vi "Acquire Pulse Result.vi"(8 "error in (no error)":errorcluster, 11 "Pulse Driver in":refnum<class "Pulse Driver.lvclass">) -> (0 "error out":errorcluster, 2 "Pulse acquired":bool, 3 "Pulse Driver out":refnum<class "Pulse Driver.lvclass">)   [LabVIEW 2021, in "Pulse Driver.lvclass"]
uses:
  Pulse Driver.lvclass
  Pulse Driver.lvclass/Pulse Driver.ctl
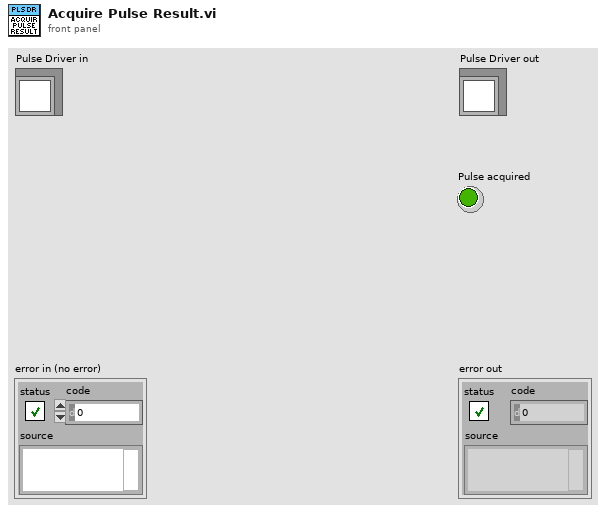
[diagram p1: front panel]
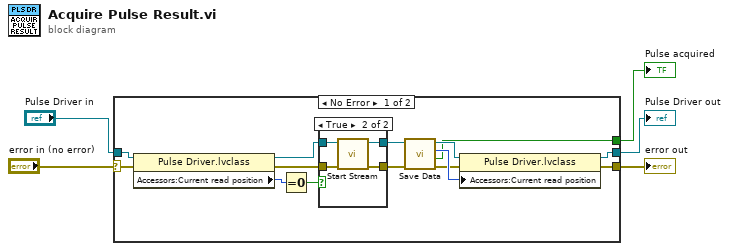
[diagram p0: block diagram]
diagram:
  n1 = case shown="No Error" "error in (no error)" {
    selector: "error in (no error)" -> [w16 w27]
    tunnel: [w8 w27] -> w4
    tunnel: [w12 w26] -> w2
    tunnel: "Pulse Driver in" -> [w15 w26]
    tunnel: [w6 _] -> w1
    frame No Error {
      n2 = property class="Pulse Driver.lvclass"(reference=w15, error in=w16) -> (reference out=w14:refnum<class "Pulse Driver.lvclass">, error out=w9:errorcluster, "Accessors:Current read position"=w7:i32)
      n3 = Equal To 0?(x=w7) -> (x = 0?=w17:bool)
      n4 = case shown="True" w17 {
        tunnel: w14 -> [w20 w24]
        tunnel: w9 -> [w21 w23]
        tunnel: [w21 w25] -> w18
        tunnel: [w20 w22] -> w19
        frame False {
        }
        frame True {
          n5 = call-dynamic "Start Stream.vi"("error in (no error)"=w23, "Pulse Driver in"=w24) -> ("error out"=w25:errorcluster, "Pulse Driver out"=w22:refnum<class "Pulse Driver.lvclass">)  [unwired: 8 in]
        }
      }
      n6 = call-dynamic "Save Data.vi"("error in (no error)"=w18, "Pulse Driver in"=w19) -> ("error out"=w10:errorcluster, "Finished"=w6:bool, "Current read position"=w11:i32, "Pulse Driver out"=w13:refnum<class "Pulse Driver.lvclass">)  [unwired: 6 in]
      n7 = property class="Pulse Driver.lvclass"(reference=w13, error in=w10, "Accessors:Current read position"=w11) -> (reference out=w12:refnum<class "Pulse Driver.lvclass">, error out=w8:errorcluster)
    }
    frame Error {
    }
  }
  "error out" <- w4
  "Pulse Driver out" <- w2
  "Pulse acquired" <- w1
